vi "Test9.vi"() -> ()   [LabVIEW 2010]
uses:
  <vilib>/MDSplus/Library/MDSplus.lvlib
panel:
  in  "Path":string=":NUMX"
  in  "Mode":string="EDIT"
  in  "Shot":i32=-1
  in  "Name":string="my_tree"
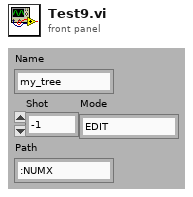
[diagram p1: front panel]
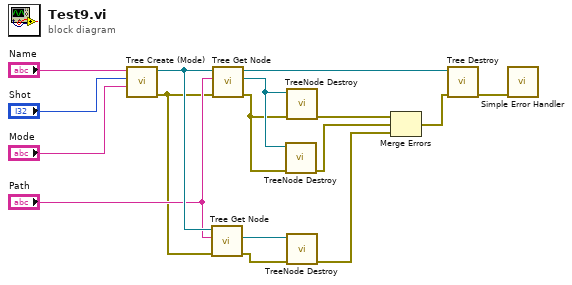
[diagram p0: block diagram]
diagram:
  n1 = call <vilib>:"Tree Create (Mode).vi"("Mode"="Mode", "Shot"="Shot", "Name"="Name") -> ("error out"=w11:errorcluster, "Tree DVR out"=w13:refnum<data-value>)  [unwired: 7 in]
  n2 = call <vilib>:"Tree Get Node.vi"("error in (no error)"=w11, "Path"="Path", "Tree DVR in"=w13) -> ("error out"=w8:errorcluster, "TreeNode DVR out"=w9:refnum<data-value>)  [unwired: 5 in, 1 out]
  n3 = call <vilib>:"Tree Get Node.vi"("error in (no error)"=w11, "Path"="Path", "Tree DVR in"=w13) -> ("error out"=w4:errorcluster, "TreeNode DVR out"=w5:refnum<data-value>, "Tree DVR out"=w10:refnum<data-value>)  [unwired: 5 in]
  n4 = call <vilib>:"TreeNode Destroy.vi"("error in (no error)"=w4, "TreeNode DVR in"=w5) -> ("error out"=w3:errorcluster)  [unwired: 8 in]
  n5 = call <vilib>:"TreeNode Destroy.vi"("error in (no error)"=w4, "TreeNode DVR in"=w5) -> ("error out"=w7:errorcluster)  [unwired: 8 in]
  n6 = call <vilib>:"TreeNode Destroy.vi"("error in (no error)"=w8, "TreeNode DVR in"=w9) -> ("error out"=w1:errorcluster)  [unwired: 8 in]
  n7 = Merge Errors(w7, w3, w1) -> (w6:errorcluster)
  n8 = call <vilib>:"Tree Destroy.vi"("error in (no error)"=w6, "Tree DVR in"=w10) -> ("error out"=w2:errorcluster)  [unwired: 8 in]
  n9 = call <vilib>:"Simple Error Handler.vi"("error in (no error)"=w2) -> ()  [unwired: 4 in, 5 out]
